vi "Average.vi"(1 "Input 3":dbl, 2 "Input 2":dbl, 3 "Input 1":dbl) -> (0 "Average":dbl)   [LabVIEW 2023]
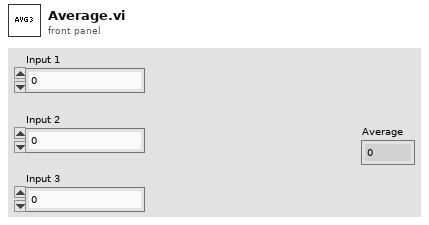
[diagram p1: front panel]
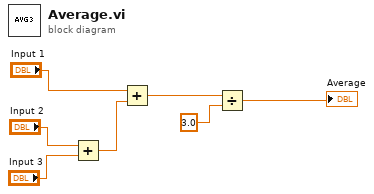
[diagram p0: block diagram]
diagram:
  n1 = Add(x="Input 2", y="Input 3") -> (x+y=w2:dbl)
  n2 = Add(x="Input 1", y=w2) -> (x+y=w4:dbl)
  n3 = Divide(x=w4, y=3.0) -> (x/y=→"Average":dbl)
